vi "kwadrat czy panorama.vi"(7 "Pane":refnum<vi>, 8 "error in (no error)":errorcluster, 11 "Array in":refnum<vi>[](array[refnum])) -> (0 "error out":errorcluster, 2 "Ulozenie":T1[](array[typedef]), 3 "Array out":refnum<vi>[](array[refnum]))   [LabVIEW 2014]
doc: "Wybiera format ułożenia obiektów\nw zakładce Konfiguracja\nw zależności od formatu monitora kwadratowy/panoramiczny"
uses:
  <vilib>/Utility/miscctls.llb/LVPositionTypeDef.ctl
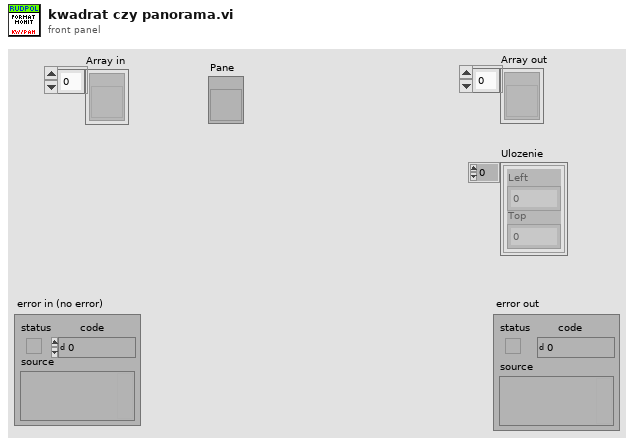
[diagram p1: front panel]
types:
  T1 = typedef "LVPositionTypeDef.ctl" = cluster{"Left":i32, "Top":i32}
  T2 = typedef "LVBoundsTypeDef.ctl" = cluster{"Width":u32, "Height":u32}
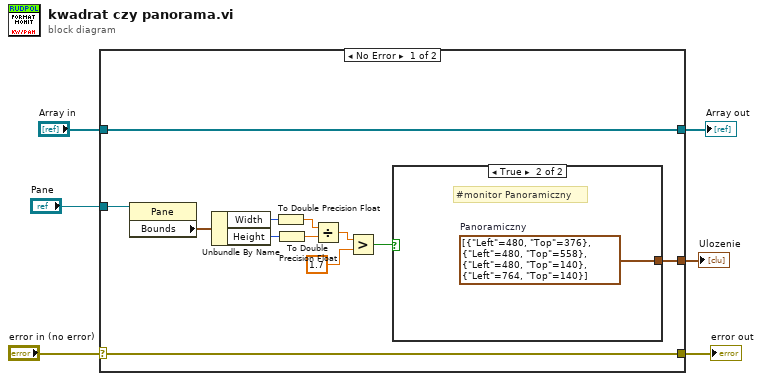
[diagram p0: block diagram]
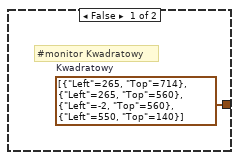
[diagram p2: hidden frame]
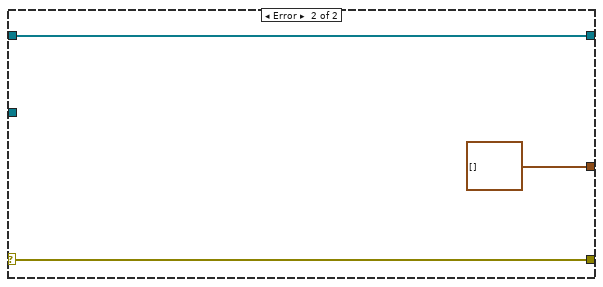
[diagram p3: hidden frame]
diagram:
  n1 = case shown="No Error" "error in (no error)" {
    selector: "error in (no error)" -> [w7 w23]
    tunnel: [w7 w23] -> w5
    tunnel: "Array in" -> [w18 w22]
    tunnel: [w18 w22] -> w3
    tunnel: [w17 T1[] [] ("Kwadratowy")] -> w2
    tunnel: "Pane" -> [w16 _]
    frame No Error {
      n2 = property class="Pane"(reference=w16) -> ("Bounds"=w15:T2)  [unwired: 1 in, 2 out]
      n3 = Unbundle By Name(w15) -> ("Width"=w14:u32, "Height"=w13:u32)
      n4 = To Double Precision Float(number=w14) -> (double precision float=w11:dbl)
      n5 = To Double Precision Float(number=w13) -> (double precision float=w12:dbl)
      n6 = Divide(x=w11, y=w12) -> (x/y=w10:dbl)
      n7 = Greater?(x=w10, y=1.7) -> (0:w8:bool)
      n8 = case shown="True" w8 {
        tunnel: [w19 w20] -> w17
        frame False {
          w19 = T1[] [{"Left"=265, "Top"=714}, {"Left"=265, "Top"=560}, {"Left"=-2, "Top"=560}, {"Left"=550, "Top"=140}]  # Kwadratowy
          # "#monitor Kwadratowy"
        }
        frame True {
          w20 = T1[] [{"Left"=480, "Top"=376}, {"Left"=480, "Top"=558}, {"Left"=480, "Top"=140}, {"Left"=764, "Top"=140}]  # Panoramiczny
          # "#monitor Panoramiczny"
        }
      }
    }
    frame Error {
    }
  }
  "error out" <- w5
  "Array out" <- w3
  "Ulozenie" <- w2
